vi "Configure Math Channel.vi"(7 "Math Function (1:Subtract)":i32(slide)=1, 8 "error in (no error)":errorcluster {"code" format="%.0x"}, 9 "Math Source 2 (\"CH2\")":string(combo)="CH2", 10 "Math Source 1 (\"CH1\")":string(combo)="CH1", 11 "VISA Resource Name":refnum<visa-resource-name>) -> (0 "error out":errorcluster {"code" format="%.0x"}, 3 "VISA Resource Name Out":refnum<visa-resource-name>)   [LabVIEW 2010, in "Tektronix TDS 3000 Series.lvlib"]
doc: "This VI configures a math channel for standard waveform math operations. These operations are inverting, adding, subtracting, multiplying, and dividing.\n\nNotes:\n\n(1) To configure a math channel to calculate an FFT, use the tktds3k Configure Math Channel FFT VI."
uses:
  <instrlib>/Tektronix TDS 3000 Series/Tektronix TDS 3000 Series.lvlib
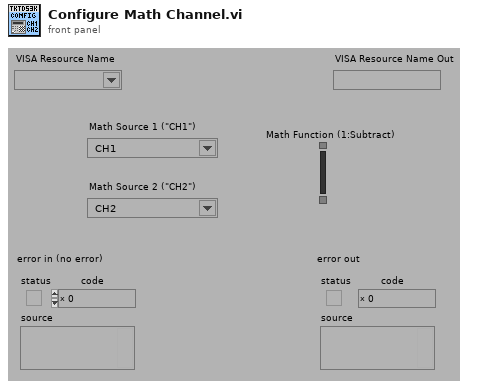
[diagram p1: front panel]
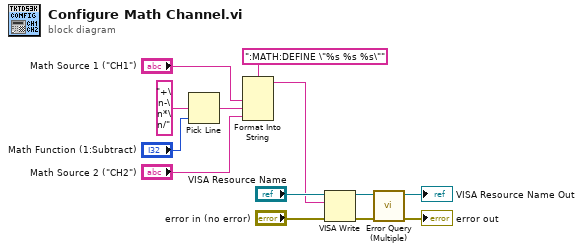
[diagram p0: block diagram]
diagram:
  n1 = Pick Line(multi-line string="+\n-\n*\n/", line index="Math Function (1:Subtract)") -> (output string=w9:string)  [unwired: 1 in]
  n2 = Format Into String(format string=":MATH:DEFINE \"%s %s %s\"", "Math Source 1 (\"CH1\")", w9, "Math Source 2 (\"CH2\")") -> (resulting string=w6:string)  [unwired: 2 in, 1 out]
  n3 = VISA Write(VISA resource name="VISA Resource Name", write buffer=w6, error in (no error)="error in (no error)") -> (VISA resource name out=w4:refnum<visa-resource-name>, error out=w3:errorcluster)  [unwired: 1 out]
  n4 = call <instrlib>:"Error Query (Multiple).vi"("error in (no error)"=w3, "VISA Resource Name"=w4) -> ("error out"=→"error out":errorcluster, "VISA Resource Name Out"=→"VISA Resource Name Out":refnum<visa-resource-name>)  [unwired: 6 in, 2 out]
